vi "Prediction.vi"(8 "Puissance Live":dbl, 11 "Puissance prédédente":dbl[](array[numeric])) -> (2 "Puissance Prédite":dbl)   [LabVIEW 2018]
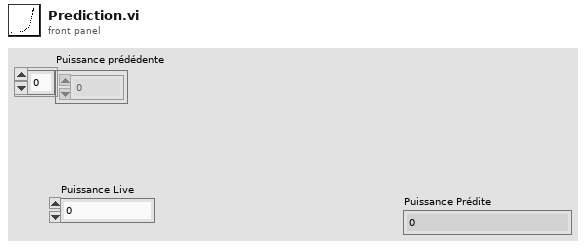
[diagram p1: front panel]
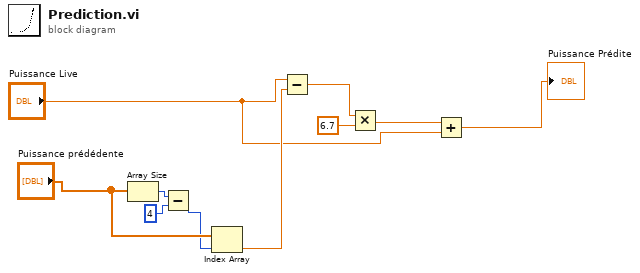
[diagram p0: block diagram]
diagram:
  n1 = Array Size(array="Puissance prédédente") -> (size(s)=w10:i32)
  n2 = Subtract(x=w10, y=4) -> (x-y=w7:i32)
  n3 = Index Array(array="Puissance prédédente", index=w7) -> (element=w2:dbl)
  n4 = Subtract(x="Puissance Live", y=w2) -> (x-y=w6:dbl)
  n5 = Multiply(x=w6, y=6.7) -> (x*y=w4:dbl)
  n6 = Add(x=w4, y="Puissance Live") -> (x+y=→"Puissance Prédite":dbl)
